vi "Read Source.vi"(8 "error in (no error)":errorcluster, 11 "Move in":refnum<class "Move.lvclass">) -> (0 "error out":errorcluster, 2 "Square":T1={"File"=enum."d", "Rank"=enum."4"}, 3 "Move out":refnum<class "Move.lvclass">)   [LabVIEW 2015, in "Chesslib.lvlib" / "Move.lvclass"]
uses:
  Move.lvclass
  typedef/Square.ctl
  typedef/File.ctl
  typedef/Rank.ctl
  Move.lvclass/Move.ctl
  Chesslib.lvlib
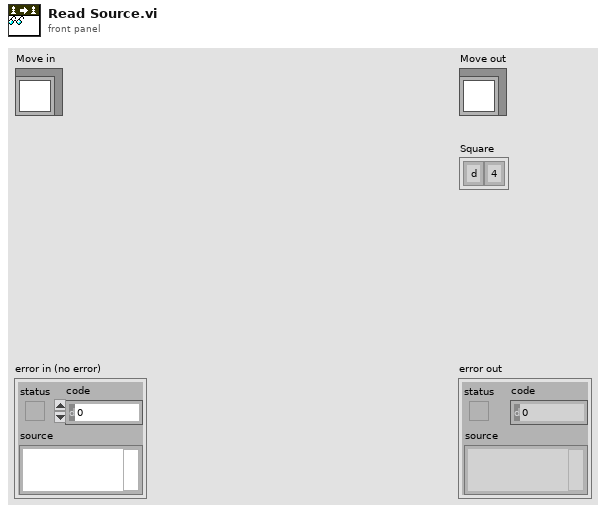
[diagram p1: front panel]
types:
  T1 = typedef "Chesslib.lvlib/Square.ctl" = cluster{"File":T2, "Rank":T3}
  T2 = typedef "Chesslib.lvlib/File.ctl" = enum8{"a", "b", "c", "d", "e", "f", "g", "h"}
  T3 = typedef "Chesslib.lvlib/Rank.ctl" = enum8{"1", "2", "3", "4", "5", "6", "7", "8"}
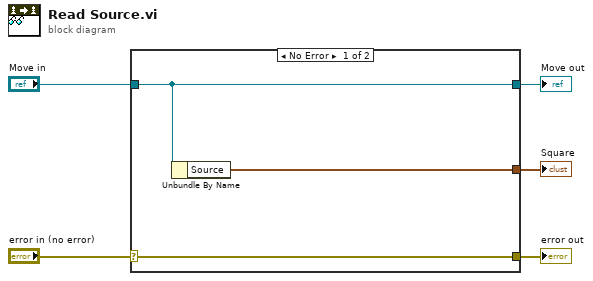
[diagram p0: block diagram]
diagram:
  n1 = case shown="No Error" "error in (no error)" {
    selector: "error in (no error)" -> [w8 w9]
    tunnel: [w8 w9] -> w4
    tunnel: [w7 w10] -> w2
    tunnel: "Move in" -> [w7 w10]
    tunnel: [w6 _] -> w1
    frame No Error {
      n2 = Unbundle By Name(w7) -> ("Source"=w6:T1)
    }
    frame Error {
    }
  }
  "error out" <- w4
  "Move out" <- w2
  "Square" <- w1
